vi "Acquire.vi"(8 "error in (no error)":cluster{"状态":bool, "代码":i32, "源":string} caption="错误输入（无错误）", 9 "数据队列":refnum<queue>, 10 "数据通知器":refnum<notifier>, 11 "硬件资源输入":T1) -> (0 "error out":cluster{"状态":bool, "代码":i32, "源":string} caption="错误输出", 3 "硬件资源输出":T1)   [LabVIEW 2012, in "Acquisition.lvlib"]
doc: "执行采集。替换程序框图的内容，添加对采集硬件的调用。"
uses:
  Acquisition.lvlib
  Hardware Configuration.ctl
  Signal Type.ctl
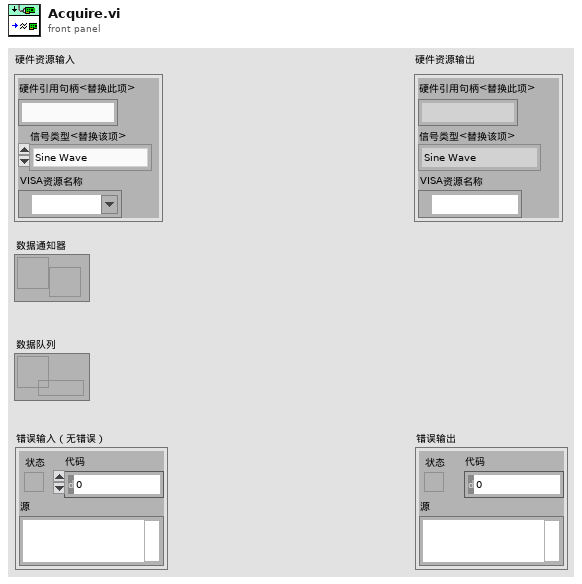
[diagram p1: front panel]
types:
  T1 = typedef "Acquisition.lvlib/Hardware Configuration.ctl" = cluster{"硬件引用句柄<替换此项>":string, "信号类型<替换该项>":T2, "VISA资源名称":refnum<visa-resource-name>}
  T2 = typedef "Acquisition.lvlib/Signal Type.ctl" = enum16{"Sine Wave", "Square with Noise"}
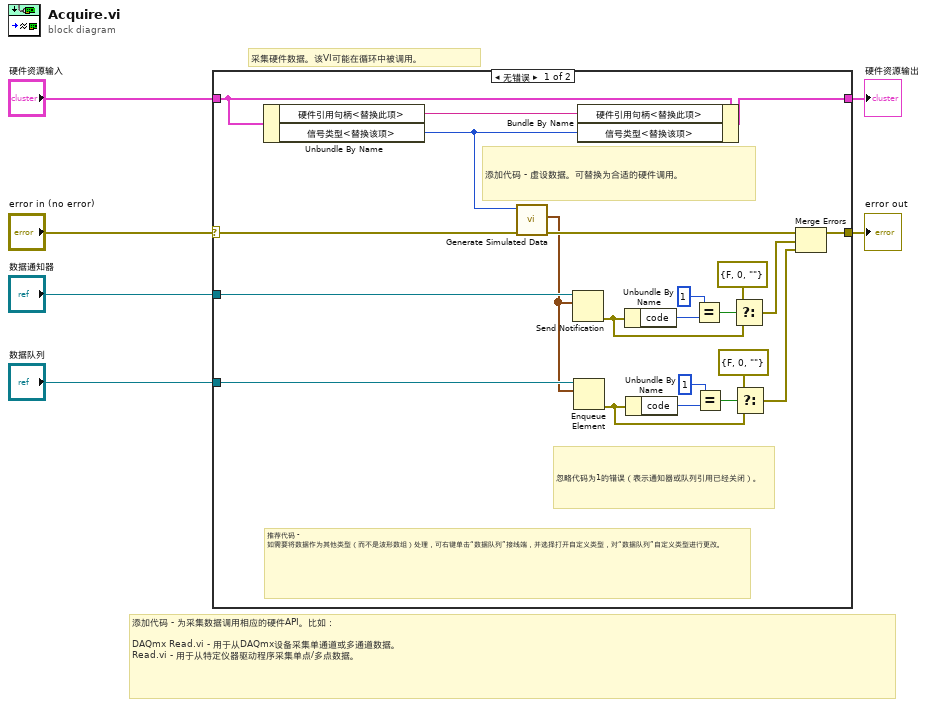
[diagram p0: block diagram]
diagram:
  # "采集硬件数据。该VI可能在循环中被调用。"
  # "添加代码 - 为采集数据调用相应的硬件API。比如：\n\nDAQmx Read.vi - 用于从DAQmx设备采集单通道或多通道数据。\nRead.vi - 用于从特定仪器驱动程序采集单点/多点数据。"
  n1 = case shown="无错误" "error in (no error)" {
    selector: "error in (no error)" -> [w26 w29]
    tunnel: [w27 w29] -> w5
    tunnel: "硬件资源输入" -> [w22 w30]
    tunnel: [w28 w30] -> w3
    tunnel: "数据通知器" -> [w21 _]
    tunnel: "数据队列" -> [w8 _]
    frame No Error {
      # "忽略代码为1的错误（表示通知器或队列引用已经关闭）。"
      # "添加代码 - 虚设数据。可替换为合适的硬件调用。"
      # "推荐代码 - 如需要将数据作为其他类型（而不是波形数组）处理，可右键单击“数据队列”接线端，并选择打开自定义类型，对“数据队列”自定义类型进行更改。"
      n2 = Unbundle By Name(w22) -> ("硬件引用句柄<替换此项>"=w23:string, "信号类型<替换该项>"=w24:T2)
      n3 = call "Generate Simulated Data.vi"("error in (no error)"=w26, "信号类型"=w24) -> ("error out"=w25:cluster{"状态":bool, "代码":i32, "源":string}, "图形数据"=w7:waveform(dbl)[])  [unwired: 7 in]
      n4 = Send Notification(notification=w7, notifier=w21) -> (error out=w17:errorcluster)  [unwired: 1 in, 1 out]
      n5 = Enqueue Element(queue=w8, element=w7) -> (error out=w13:errorcluster)  [unwired: 2 in, 2 out]
      n6 = Bundle By Name(cluster=w22, "硬件引用句柄<替换此项>"=w23, "信号类型<替换该项>"=w24) -> (w28:T1)
      n7 = Unbundle By Name(w17) -> ("code"=w20:i32)
      n8 = Unbundle By Name(w13) -> ("code"=w10:i32)
      n9 = Equal?(x=1, y=w20) -> (x = y?=w18:bool)
      n10 = Equal?(x=1, y=w10) -> (x = y?=w12:bool)
      n11 = Select(t=errorcluster {"status"=FALSE, "code"=0, "source"=""} ("error constant"), s=w18, f=w17) -> (s? t:f=w16:errorcluster)
      n12 = Select(t=errorcluster {"status"=FALSE, "code"=0, "source"=""} ("error constant"), s=w12, f=w13) -> (s? t:f=w9:errorcluster)
      n13 = Merge Errors(w25, w16, w9) -> (w27:errorcluster)
    }
    frame Error {
    }
  }
  "硬件资源输出" <- w3
  "error out" <- w5
